vi "ExeSqlQuery.vi"(8 "error in (no error)":errorcluster, 10 "SqlQuery":string, 11 "TMflexDatabase in":refnum<class "TMflexDatabase.lvclass">) -> (0 "error out":errorcluster, 2 "data":variant[][](array[variant]), 3 "TMflexDatabase out":refnum<class "TMflexDatabase.lvclass">)   [LabVIEW 2015, in "TMflexDatabase.lvclass"]
uses:
  TMflexDatabase.lvclass
  TMflexDatabase.lvclass/TMflexDatabase.ctl
  <vilib>/addons/database/Connection.llb/DB Tools Open Connec (String).vi
  <vilib>/addons/database/Connection.llb/Conn Execute.vi
  <vilib>/addons/database/Recordset.llb/Rec Fetch Recordset Data (R).vi
  <vilib>/addons/database/Recordset.llb/Rec Destroy - Connection.vi
  <vilib>/addons/database/NI_Database_API.lvlib
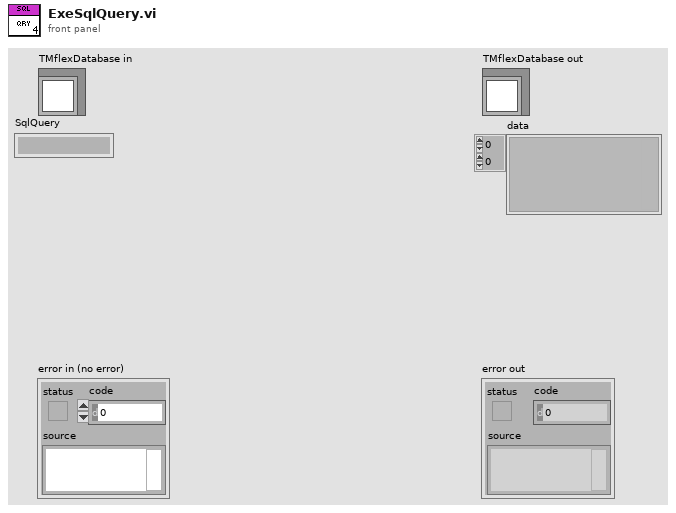
[diagram p1: front panel]
types:
  T1 = typedef "NI_Database_API.lvlib/Conn ObjectReference.ctl" = refnum<k1>
  T2 = typedef "NI_Database_API.lvlib/Rec ObjectReference.ctl" = refnum<k1>
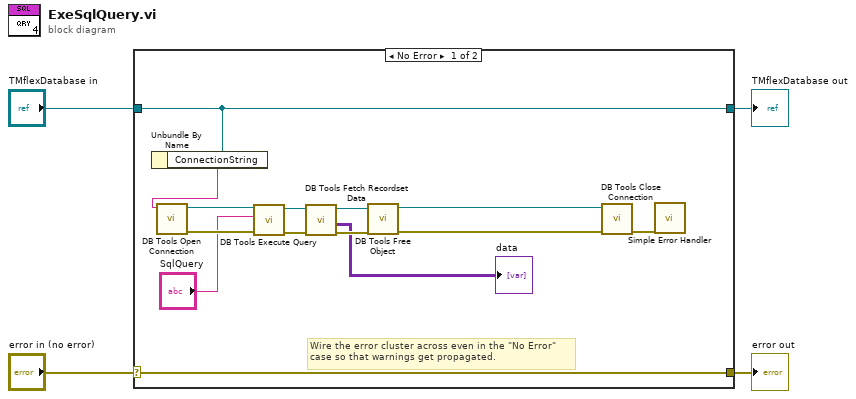
[diagram p0: block diagram]
diagram:
  n1 = case shown="No Error" "error in (no error)" {
    selector: "error in (no error)" -> [w17 w19]
    tunnel: [w17 w19] -> w3
    tunnel: [w13 w18] -> w1
    tunnel: "TMflexDatabase in" -> [w13 w18]
    frame No Error {
      # "Wire the error cluster across even in the \"No Error\"\ncase so that warnings get propagated."
      n2 = Unbundle By Name(w13) -> ("ConnectionString"=w12:string)
      n3 = call-poly <vilib>:"DB Tools Open Connection.vi"("connection information"=w12) -> ("error out"=w15:errorcluster, "connection reference"=w14:T1)  [unwired: 7 in]
      n4 = call-poly <vilib>:"DB Tools Execute Query.vi"("error in (no error)"=w15, "SQL query"="SqlQuery", "connection reference"=w14) -> ("error out"=w10:errorcluster, "recordset reference"=w8:T2)  [unwired: 5 in]
      n5 = call-poly <vilib>:"DB Tools Fetch Recordset Data.vi"("recordset reference"=w8) -> ("recordset data"=→"data":variant[][], "recordset reference out"=w7:T2)  [unwired: 4 in, 1 out]
      n6 = call-poly <vilib>:"DB Tools Free Object.vi"("error in (no error)"=w10, "recordset reference"=w7) -> ("error out"=w9:errorcluster, "connection reference"=w5:T1)  [unwired: 8 in]
      n7 = call <vilib>:"DB Tools Close Connection.vi"("error in (no error)"=w9, "connection reference"=w5) -> ("error out"=w16:errorcluster)  [unwired: 5 in]
      n8 = call <vilib>:"Simple Error Handler.vi"("error in (no error)"=w16) -> ()  [unwired: 4 in, 5 out]
    }
    frame Error {
    }
  }
  "error out" <- w3
  "TMflexDatabase out" <- w1
